vi "Configure Alarm Delay IO.vi"(0 "VISA resource name":refnum<visa-resource-name>, 5 "Channel (0001)":string="0001", 7 "Alarm Delay Time":cluster{"Hour":i32, "Min":i32, "Sec":i32}={"Hour"=0, "Min"=0, "Sec"=10} {"Sec" min=0 max=59; "Min" min=0 max=59; "Hour" min=0 max=24}, 11 "error in (no error)":errorcluster) -> (4 "VISA resource name out":refnum<visa-resource-name>, 6 "Channel":string, 15 "error out":errorcluster)   [LabVIEW 2020, in "Yokogawa GX Series.lvlib"]
doc: "Sets the alarm delay time for IO channels.\n\nCommands: SAlmDlyIO"
uses:
  <instrlib>/Yokogawa GX Series/Yokogawa GX Series.lvlib
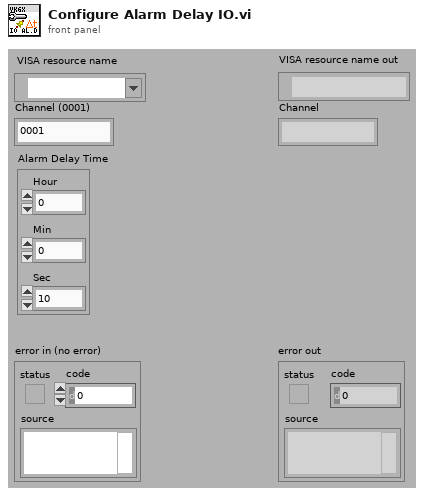
[diagram p1: front panel]
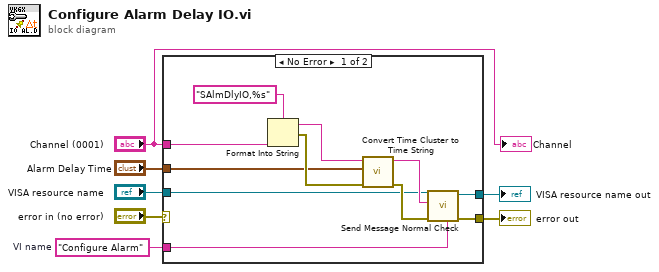
[diagram p0: block diagram]
diagram:
  w7 = "Configure Alarm"  # VI name
  n1 = case shown="No Error" "error in (no error)" {
    selector: "error in (no error)" -> [_ w19]
    tunnel: w7 -> [w18 _]
    tunnel: [w17 w20] -> w6
    tunnel: [w16 w19] -> w5
    tunnel: "VISA resource name" -> [w10 w20]
    tunnel: "Alarm Delay Time" -> [w9 _]
    tunnel: "Channel (0001)" -> [w8 _]
    frame No Error {
      n2 = Format Into String(format string="SAlmDlyIO,%s" ("形式文字列"), w8) -> (resulting string=w13:string, error out=w14:errorcluster)  [unwired: 2 in]
      n3 = call <instrlib>:"Convert Time Cluster to Time String.vi"("error in (no error)"=w14, "Time"=w9, "String"=w13) -> ("error out"=w11:errorcluster, "Time String"=w12:string)  [unwired: 7 in]
      n4 = call <instrlib>:"Send Message Normal Check.vi"("Source (\"\")"=w18, "error in (no error)"=w11, "Send Message (\"\")"=w12, "VISA resource name"=w10) -> ("error out"=w16:errorcluster, "VISA resource name out"=w17:refnum<visa-resource-name>)  [unwired: 2 in, 4 out]
    }
    frame Error {
    }
  }
  "error out" <- w5
  "VISA resource name out" <- w6
  "Channel" <- "Channel (0001)"
